vi "pair modules.vi"(6 "paired engine in":refnum<class "engine configuration.lvclass">, 8 "error in":errorcluster, 9 "engine configuration in":refnum<class "engine configuration.lvclass">, 10 "module to pair with":refnum<class "TEC editor node.lvclass">, 11 "UDP Broadcast Editor Node in":refnum<class "TEC editor node.lvclass">) -> (0 "error out":errorcluster, 1 "engine configuration out":refnum<class "engine configuration.lvclass">, 2 "module to pair with out":refnum<class "TEC editor node.lvclass">, 3 "UDP Broadcast Editor Node out":refnum<class "TEC editor node.lvclass">, 4 "paired engine out":refnum<class "engine configuration.lvclass">)   [LabVIEW 2013, in "TEC editor node.lvclass"]
uses:
  TEC editor node.lvclass
  <vilib>/NI/Module Execution Interface/Engine Configuration/engine configuration.lvclass
  TEC editor node.lvclass/TEC editor node.ctl
  <vilib>/NI/Configuration Framework/serializable configuration/NISE_CEF_serializable configuration.lvclass/NISE_CEF_serializable configuration.ctl
  <vilib>/NI/Configuration Framework/serializable configuration/NISE_CEF_serializable configuration.lvclass
  configuration/TEC configuration.lvclass
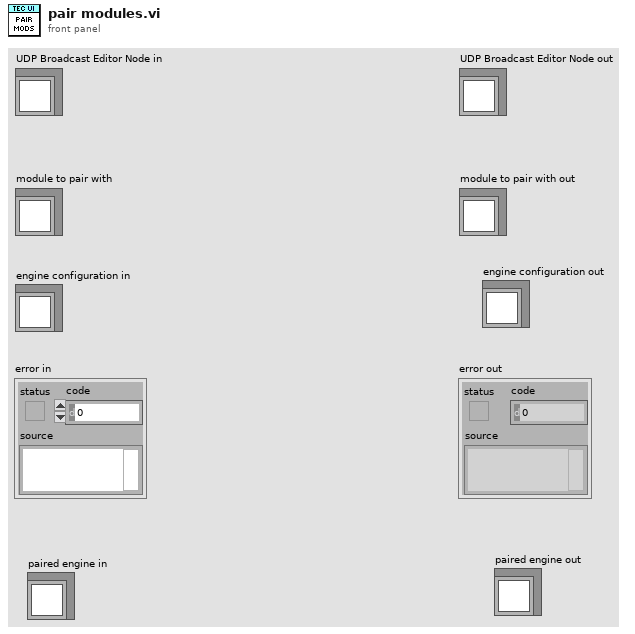
[diagram p1: front panel]
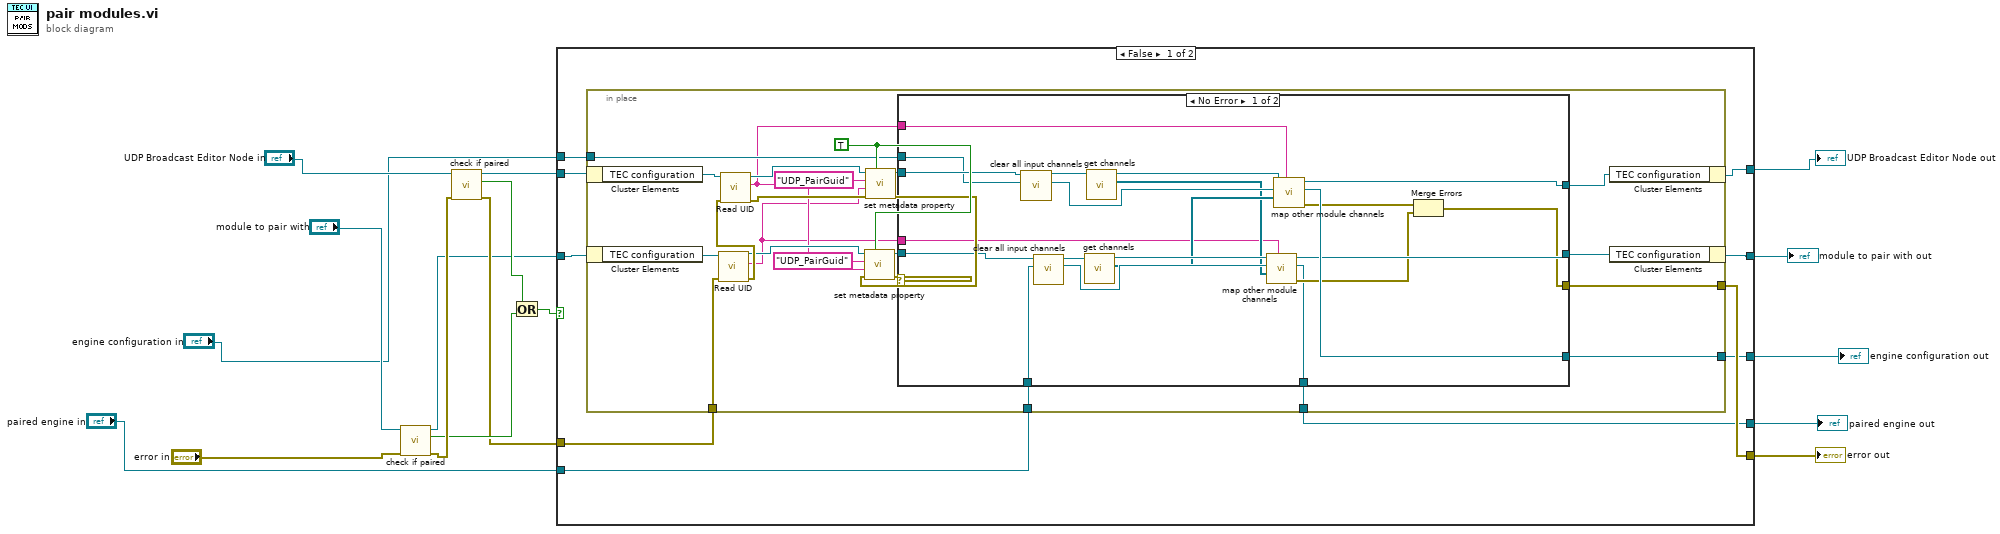
[diagram p0: block diagram]
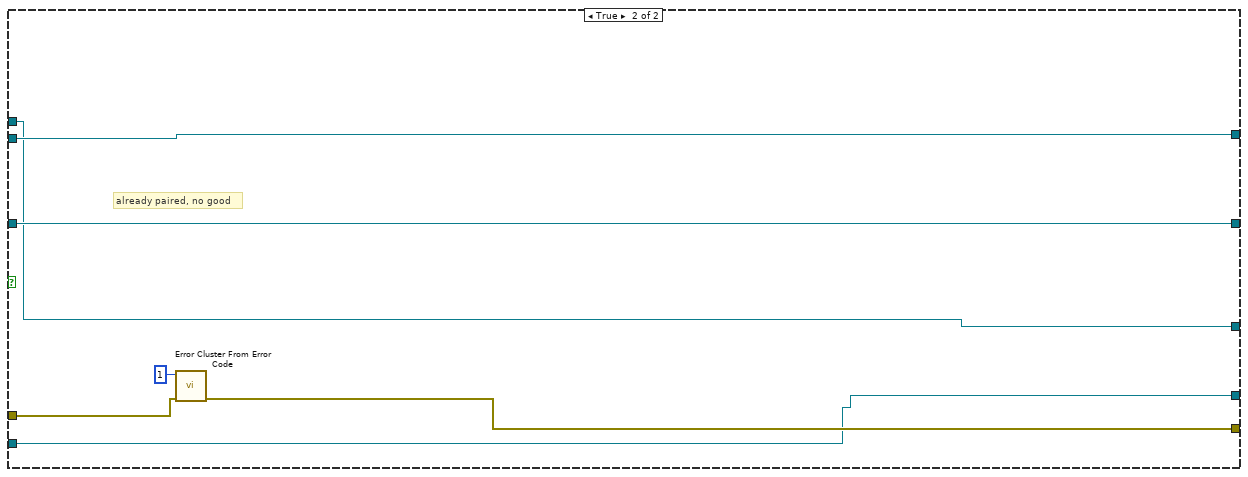
[diagram p3: hidden frame]
diagram:
  n1 = call "check if paired.vi"("error in"="error in", "UDP Broadcast Editor Node in"="module to pair with") -> ("error out"=w14:errorcluster, "paired"=w12:bool, "UDP Broadcast Editor Node out"=w6:refnum<class "TEC editor node.lvclass">)  [unwired: 7 in]
  n2 = call "check if paired.vi"("error in"=w14, "UDP Broadcast Editor Node in"="UDP Broadcast Editor Node in") -> ("error out"=w10:errorcluster, "paired"=w13:bool, "UDP Broadcast Editor Node out"=w7:refnum<class "TEC editor node.lvclass">)  [unwired: 7 in]
  n3 = Or(x=w13, y=w12) -> (x .or. y?=w11:bool)
  n4 = case shown="False" w11 {
    tunnel: w10 -> [w24 w83]
    tunnel: [w23 w81] -> w9
    tunnel: [w26 w80] -> w8
    tunnel: w7 -> [w27 w80]
    tunnel: w6 -> [w25 w79]
    tunnel: [w22 w79] -> w5
    tunnel: "engine configuration in" -> [w21 w78]
    tunnel: "paired engine in" -> [w20 w77]
    tunnel: [w19 w78] -> w2
    tunnel: [w18 w77] -> w1
    frame False {
      n5 = in-place {
        in-place-border: w24 -> [w48]
        in-place-border: [w38] -> w23
        in-place-border: w21 -> [w33]
        in-place-border: w20 -> [w32]
        in-place-border: [w30] -> w19
        in-place-border: [w29] -> w18
        w44 = TRUE ("overwrite?")
        n6 = in-place-cluster #1(w27) -> ("TEC configuration"=w50:refnum<class "TEC configuration.lvclass">)
        n7 = in-place-cluster #2(w25) -> ("TEC configuration"=w49:refnum<class "TEC configuration.lvclass">)
        n8 = call <vilib>:"Read UID.vi"("error in"=w48, "configuration in"=w49) -> ("error out"=w47:errorcluster, "instance id"=w28:string, "configuration out"=w42:refnum<class "TEC configuration.lvclass">)  [unwired: 7 in]
        n9 = call <vilib>:"Read UID.vi"("error in"=w47, "configuration in"=w50) -> ("error out"=w41:errorcluster, "instance id"=w31:string, "configuration out"=w43:refnum<class "TEC configuration.lvclass">)  [unwired: 7 in]
        n10 = call <vilib>:"set metadata property.vi"("overwrite?"=w44, "error in"=w41, "value"=w28, "key"="UDP_PairGuid", "configuration in"=w43) -> ("error out"=w40:errorcluster, "configuration out"=w34:refnum<class "TEC configuration.lvclass">)  [unwired: 5 in]
        n11 = call <vilib>:"set metadata property.vi"("overwrite?"=w44, "error in"=w40, "value"=w31, "key"="UDP_PairGuid", "configuration in"=w42) -> ("error out"=w39:errorcluster, "configuration out"=w37:refnum<class "TEC configuration.lvclass">)  [unwired: 5 in]
        n12 = case shown="No Error" w39 {
          selector: w39 -> [_ w76]
          tunnel: [w57 w76] -> w38
          tunnel: w37 -> [w71 w75]
          tunnel: [w58 w75] -> w36
          tunnel: [w63 w74] -> w35
          tunnel: w34 -> [w70 w74]
          tunnel: w33 -> [w67 w72]
          tunnel: w32 -> [w65 w73]
          tunnel: w31 -> [w60 _]
          tunnel: [w62 w72] -> w30
          tunnel: [w55 w73] -> w29
          tunnel: w28 -> [w51 _]
          frame No Error {
            n13 = call "clear all input channels.vi"("engine configuration in"=w67, "TEC configuration in"=w70) -> ("engine configuration out"=w66:refnum<class "engine configuration.lvclass">, "TEC configuration out"=w69:refnum<class "TEC configuration.lvclass">)  [unwired: 8 in]
            n14 = call "clear all input channels.vi"("engine configuration in"=w65, "TEC configuration in"=w71) -> ("engine configuration out"=w54:refnum<class "engine configuration.lvclass">, "TEC configuration out"=w68:refnum<class "TEC configuration.lvclass">)  [unwired: 8 in]
            n15 = call-dynamic "get channels.vi"("TEC configuration in"=w68) -> ("channels"=w53:refnum<class "TBM channel.lvclass">[], "TEC configuration out"=w59:refnum<class "TEC configuration.lvclass">)  [unwired: 9 in]
            n16 = call-dynamic "get channels.vi"("TEC configuration in"=w69) -> ("channels"=w52:refnum<class "TBM channel.lvclass">[], "TEC configuration out"=w64:refnum<class "TEC configuration.lvclass">)  [unwired: 9 in]
            n17 = call "map other module channels.vi"("instance id"=w51, "channels"=w52, "engine configuration in"=w54, "TEC configuration in"=w59) -> ("error out"=w56:errorcluster, "engine configuration out"=w55:refnum<class "engine configuration.lvclass">, "TEC configuration out"=w58:refnum<class "TEC configuration.lvclass">)  [unwired: 5 in]
            n18 = call "map other module channels.vi"("instance id"=w60, "channels"=w53, "engine configuration in"=w66, "TEC configuration in"=w64) -> ("error out"=w61:errorcluster, "engine configuration out"=w62:refnum<class "engine configuration.lvclass">, "TEC configuration out"=w63:refnum<class "TEC configuration.lvclass">)  [unwired: 5 in]
            n19 = Merge Errors(w61, w56) -> (w57:errorcluster)
          }
          frame Error {
          }
        }
        n20 = in-place-cluster #1("TEC configuration"=w35) -> (w26:refnum<class "TEC editor node.lvclass">)
        n21 = in-place-cluster #2("TEC configuration"=w36) -> (w22:refnum<class "TEC editor node.lvclass">)
      }
    }
    frame True {
      # "already paired, no good"
      n22 = call <vilib>:"Error Cluster From Error Code.vi"("error in (no error)"=w83, "error code (0)"=1) -> ("error out"=w81:errorcluster)  [unwired: 7 in]
    }
  }
  "error out" <- w9
  "UDP Broadcast Editor Node out" <- w8
  "module to pair with out" <- w5
  "engine configuration out" <- w2
  "paired engine out" <- w1
